vi "Boolean to Enable-Disabled.vi"(0 "Enabled?":bool, 1 "Invert?  (Default: False)":bool) -> (2 "Disabled State":T1(ring))   [LabVIEW 2020, in "AR Example.lvlib"]
uses:
  AR Example.lvlib
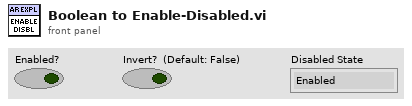
[diagram p1: front panel]
types:
  T1 = enum8{"Enabled", "Disabled", "Disabled and Grayed Out"}
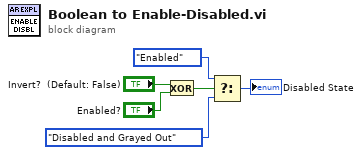
[diagram p0: block diagram]
diagram:
  n1 = Exclusive Or(1:"Enabled?", 2:"Invert?  (Default: False)") -> (0:w2:bool)
  n2 = Select(t=T1."Enabled" ("Disabled"), s=w2, f=T1."Disabled and Grayed Out") -> (s? t:f=→"Disabled State":T1)
